vi "CsTool-GetSystemFill.vi"(2 "Index (0)":i16 min=0 max=64 step=1, 3 "Sample Bits (0)":u32 max=5 step=1, 4 "Channel Count (0)":u32 max=64 step=1, 5 "Board Name (Any)":string="any") -> (0 "Error Code":i32, 1 "Handle Cluster":T1)   [LabVIEW 2022 SP3]
doc: "This VI returns a unique Handle Cluster for an available CompuScope system. This Handle Cluster is used as an input to most other CsTool VIs. The Board Type, Channel Count, Sample Bits, and Index input fields may be used to search only for CompuScope systems with capabilities specified in these input fields. An \"any\" in the Board Type field will cause the VI to search for any CompuScope model and return the Handle Cluster for the first available CompuScope system. Similarly, a 0 in any of the numerical fields means that the VI will not narrow its search using this field. If all fields are \"any\" or 0, the VI returns the Handle Cluster for the first available CompuScope system. The Index input may be used to select a specific CompuScope system by ordinal number. \n\nIf the call is successful, a 1 is returned in the Error Code indicator and a valid Handle Cluster is returned as the Handle Cluster output. \n\nIf the call is unsuccessful, and if the Index input is zero, all CompuScope handles that were allocated within LabVIEW will be freed. The VI will then attempt to obtain a CompuScope system handle again. This procedure of freeing all CompuScope system handles and re-attempting to obtain a handle is done in order to recover from cases where VI operation was aborted without correctly freeing associated handles. If this second attempt also fails, a zero is returned in the Handle Cluster field and an appropriate error code is returned in the Error Code indicator. A descriptive error string may be obtained by using CsTool-ErrorHandler.vi.\n\n\nValid Input Parameters:\n\nBoard Name (Default = Any for \"not specified\"): \nA value of \"Any\" means the board is not specified and the VI will find the first available system. To have the VI look for a specific CompuScope board, use the Board Name (e.g. CS82G, CS14200, CSVS8, etc.).\n\nChannel Count (Default = 0 for \"not specified\") \n 0\n 1\n 2\n ,...\n\nSample Bits (Default = 0 for \"not specified\"):\n 0\n 8\n 12\n 14\n 16\n 32\n\nIndex (Default = 0 for \"not specified\"):\n 0\n 1\n 2\n ,...\n\nThe Handle Cluster that is returned uniquely identifies the CompuScope system and is used in most subsequent calls to CsTool VIs. The Handle Cluster includes the Handle variable, which is an integer value that is used as the CompuScope system handle for calls to CsLv VIs. The Handle Cluster also contains the Sample Size, the sample Resolution, the sample Offset, the number of Channels and number of Boards for the system. The Sample Size is the size of one data sample in bytes. Offset is the value that represents 0 Volts. Resolution is the number of levels between 0 and full scale, or between negative full scale and 0. Resolution and Offset may be used to convert raw ADC CompuScope data into voltage values, as described in the CompuScope SDK for LabVIEW manual. \nPlease note that the Sample Size, Resolution and Offset returned in the Handle Cluster apply for the CompuScope system when it uses standard on-board firmware. Optional CompuScope firmware may change these values. For more information, see CsTool QueryAcquisitionParameters.vi."
panel:
  out "Numeric":u32
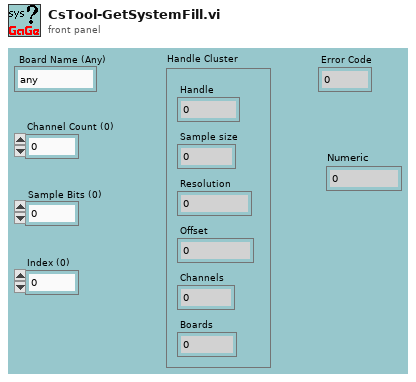
[diagram p1: front panel]
types:
  T1 = cluster{"Handle":u32, "Sample size":u32, "Resolution":i32, "Offset":i32, "Channels":u32, "Boards":u32}
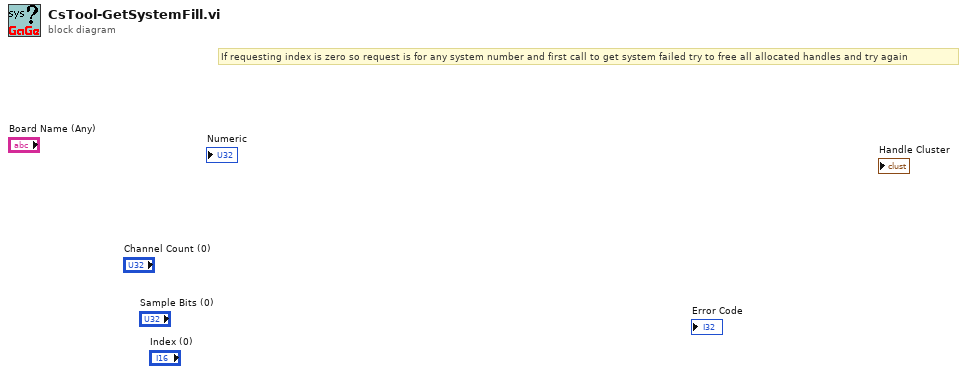
[diagram p0: block diagram]
diagram:
  # "If requesting index is zero so request is for any system number and first call to get system failed try to free all allocated handles and try again"
